vi "IPFPSGL.vi"(3 "Number":sgl) -> (0 "Fractional part":sgl, 1 "Integer part":sgl)   [LabVIEW 2017, in "GPNumeric.lvlib"]
doc: "Splits floating point <B>Number</B> into <B>Integer part</B> and <B>Fractional part</B>.\n\nThis VI is inlined.\n\nSteen Schmidt\nGPower\n16/5 2014"
uses:
  GPNumeric.lvlib
panel:
  # "Copyright © 2014\nGPower\nSee enclosed license file for terms and conditions"
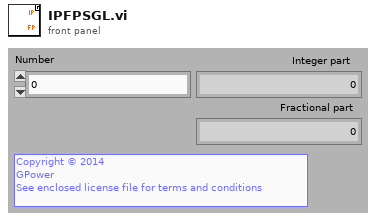
[diagram p1: front panel]
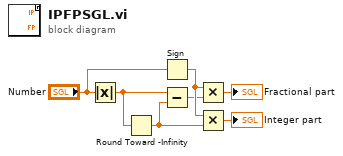
[diagram p0: block diagram]
diagram:
  n1 = Absolute Value(x="Number") -> (abs(x)=w6:sgl)
  n2 = Round Toward -Infinity(1:w6) -> (0:w5:sgl)
  n3 = Sign(1:"Number") -> (0:w7:sgl)
  n4 = Subtract(x=w6, y=w5) -> (x-y=w4:sgl)
  n5 = Multiply(x=w7, y=w4) -> (x*y=→"Fractional part":sgl)
  n6 = Multiply(x=w7, y=w5) -> (x*y=→"Integer part":sgl)
